vi "Test_RouteGuide_ResponseStreaming.vi"() -> (0 "Array of Error Description":T1)   [LabVIEW 2025]
uses:
  gRPC_ATS/TestUtility/utility.llb/array of error description.ctl
  gRPC_ATS/TestUtility/utility.llb/error description.ctl
  gRPC_ATS/TestUtility/utility.llb/error type.ctl
  examples/route_guide/route_guide_client/RPC Messages/routeguide_Feature.ctl
  examples/route_guide/route_guide_client/RPC Messages/routeguide_Point.ctl
  examples/route_guide/route_guide_client/route_guide_client.lvlib
panel:
  out "Pass":bool
  in  "Client VI Path":path=path "../../examples/route_guide/route_guide_client/ResponseStreaming RouteGuide Test.vi"
  in  "Server VI path":path=path "../../examples/route_guide/route_guide_server/Run Service.vi"
  in  "error in":errorcluster
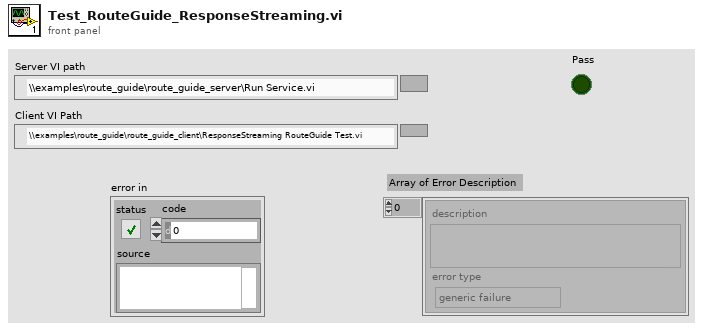
[diagram p1: front panel]
types:
  T1 = typedef "array of error description.ctl" = T2[]
  T2 = typedef "error description.ctl" = cluster{"description":string, "error type":T3}
  T3 = typedef "error type.ctl" = enum32{"generic failure", "boundary case", "precision", "expected error"}
  T4 = typedef "route_guide_client.lvlib/routeguide_Feature.ctl" = cluster{"name":string, "location":T5}
  T5 = typedef "route_guide_client.lvlib/routeguide_Point.ctl" = cluster{"latitude":i32, "longitude":i32}
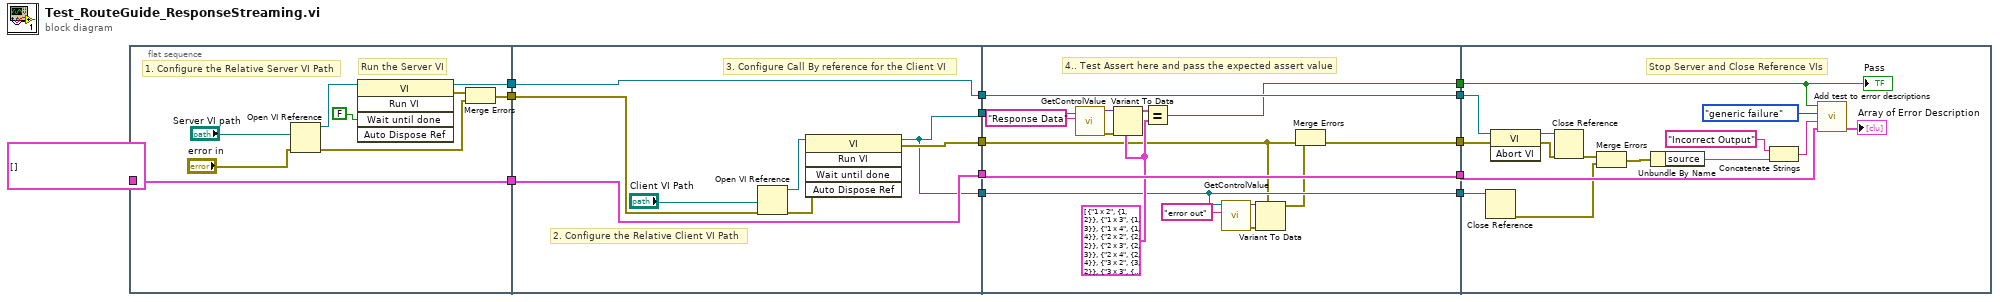
[diagram p0: block diagram]
diagram:
  n1 = flat-sequence {
    tunnel: T1 [] ("error descriptions in") -> [w19]
    tunnel: [w19] -> w14
    tunnel: [w18] -> w13
    tunnel: [w15] -> w12
    tunnel: w14 -> [w30]
    tunnel: [w30] -> w11
    tunnel: [w25] -> w10
    tunnel: [w29] -> w9
    tunnel: w13 -> [w29]
    tunnel: w12 -> [w28]
    tunnel: [w24] -> w4
    tunnel: [w24] -> w2
    tunnel: w11 -> [w47]
    tunnel: [w47] -> w8
    tunnel: w10 -> [w32]
    tunnel: [w46] -> w7
    tunnel: w9 -> [w46]
    tunnel: [w45] -> w5
    tunnel: w4 -> [w38]
    tunnel: [w38] -> w3
    tunnel: w2 -> [w44]
    tunnel: [w33] -> w1
    tunnel: w8 -> [w57]
    tunnel: w7 -> [w54]
    tunnel: w5 -> [w52]
    tunnel: w3 -> [w51]
    tunnel: w1 -> [w53]
    frame #0 {
      # "1. Configure the Relative Server VI Path"
      # "Run the Server VI"
      n2 = Open VI Reference(vi path="Server VI path", error in (no error)="error in") -> (vi reference=w21:refnum<vi>, error out=w17:errorcluster)  [unwired: 4 in]
      n3 = invoke class="VI" method="Run VI"(reference=w21, "Wait until done"=FALSE ("Wait Until Done")) -> (reference out=w18:refnum<vi>, error out=w16:errorcluster)  [unwired: 3 in, 3 out]
      n4 = Merge Errors(w16, w17) -> (w15:errorcluster)
    }
    frame #1 {
      # "2. Configure the Relative Client VI Path"
      # "3. Configure Call By reference for the Client VI"
      n5 = Open VI Reference(vi path="Client VI Path", error in (no error)=w28) -> (vi reference=w26:refnum<vi>, error out=w27:errorcluster)  [unwired: 4 in]
      n6 = invoke class="VI" method="Run VI"(reference=w26, error in=w27) -> (reference out=w24:refnum<vi>, error out=w25:errorcluster)  [unwired: 3 in, 3 out]
    }
    frame #2 {
      w40 = T4[] [{"name"="1 x 2", "location"={"latitude"=1, "longitude"=2}}, {"name"="1 x 3", "location"={"latitude"=1, "longitude"=3}}, {"name"="1 x 4", "location"={"latitude"=1, "longitude"=4}}, {"name"="2 x 2", "location"={"latitude"=2, "longitude"=2}}, {"name"="2 x 3", "location"={"latitude"=2, "longitude"=3}}, {"name"="2 x 4", "location"={"latitude"=2, "longitude"=4}}, {"name"="3 x 2", "location"={"latitude"=3, "longitude"=2}}, {"name"="3 x 3", "location"={"latitude"=3, "longitude"=3}}, {"name"="3 x 4", "location"={"latitude"=3, "longitude"=4}}] ("Response Data")
      # "4.. Test Assert here and pass the expected assert value"
      n7 = call "GetControlValue.vi"("Control Label"="Response Data", "VI Reference"=w44) -> ("error out"=w42:errorcluster, "Value"=w41:variant)  [unwired: 8 in]
      n8 = Variant To Data(error in=w42, type=w40, Variant=w41) -> (data=w39:T4[])  [unwired: 1 out]
      n9 = Equal?(x=w39, y=w40) -> (x = y?=w45:bool)
      n10 = call "GetControlValue.vi"("Control Label"="error out", "VI Reference"=w38) -> ("error out"=w36:errorcluster, "Value"=w35:variant)  [unwired: 8 in]
      n11 = Variant To Data(error in=w36, type=w32, Variant=w35) -> (data=w34:errorcluster)  [unwired: 1 out]
      n12 = Merge Errors(w34, w32) -> (w33:errorcluster)
    }
    frame #3 {
      # "Stop Server and Close Reference VIs"
      n13 = Close Reference(reference=w51) -> (error out=w49:errorcluster)  [unwired: 1 in]
      n14 = invoke class="VI" method="Abort VI"(reference=w54, error in=w53) -> (reference out=w55:refnum<vi>, error out=w56:errorcluster)  [unwired: 1 in, 1 out]
      n15 = Close Reference(reference=w55, error in (no error)=w56) -> (error out=w50:errorcluster)
      n16 = Merge Errors(w50, w49) -> (w48:errorcluster)
      n17 = Unbundle By Name(w48) -> ("source"=w59:string)
      n18 = Concatenate Strings("Incorrect Output" ("string"), w59) -> (w60:string)
      n19 = call "Add test to error descriptions.vi"("error descriptions in"=w57, "error string"=w60, "error type"=error_type."generic failure", "pass"=w52) -> ("error description out"=→"Array of Error Description":T1)  [unwired: 3 in]
      "Pass" <- w52
    }
  }
